vi "Write Check again delay.vi"(8 "error in (no error)":errorcluster, 10 "Check again delay":i32=10, 11 "Worker in":refnum<class "Worker Actor.lvclass">) -> (0 "error out":errorcluster, 3 "Worker out":refnum<class "Worker Actor.lvclass">)   [LabVIEW 2021, in "Worker Actor.lvclass"]
uses:
  Worker Actor.lvclass
  Worker Actor.lvclass/Worker Actor.ctl
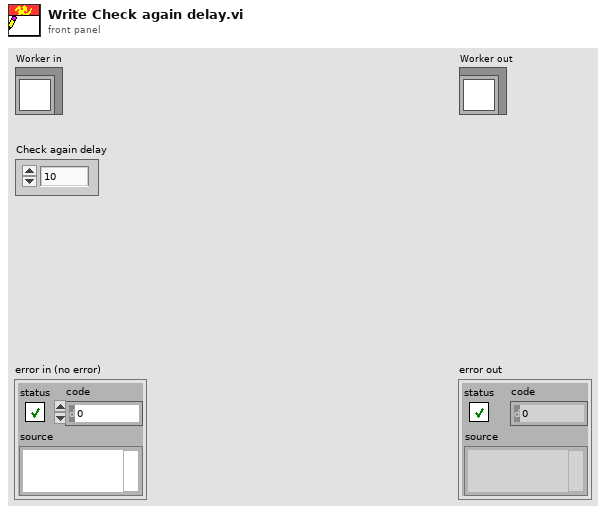
[diagram p1: front panel]
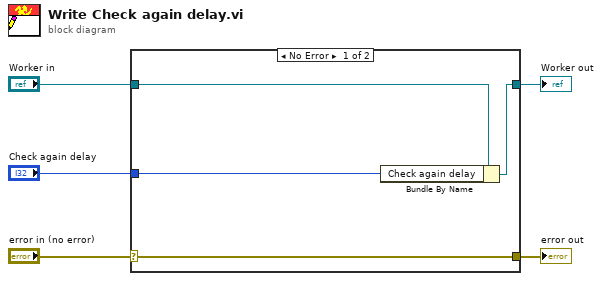
[diagram p0: block diagram]
diagram:
  n1 = case shown="No Error" "error in (no error)" {
    selector: "error in (no error)" -> [w9 w10]
    tunnel: [w9 w10] -> w4
    tunnel: [w7 w11] -> w2
    tunnel: "Worker in" -> [w8 w11]
    tunnel: "Check again delay" -> [w6 _]
    frame No Error {
      n2 = Bundle By Name(cluster=w8, "Check again delay"=w6) -> (w7:refnum<class "Worker Actor.lvclass">)
    }
    frame Error {
    }
  }
  "error out" <- w4
  "Worker out" <- w2
